vi "Rename Item Name.vi"(8 "error in (no error)":errorcluster, 9 "ForceRename?(F)":bool, 10 "New Name":string, 11 "Item Reference in":T1 format="%.0x") -> (0 "error out":errorcluster, 2 "Request invalid?":bool, 3 "Item Reference out":T1 format="%.0x")   [LabVIEW 2013, in "Hierarchy Framework.lvlib" / "Item.lvclass"]
doc: "Applies a <B>New Name</B> to the item specified by <B>Item Reference in</B>. If the <B>New Name</B> you specify already exists in the same section, this VI does nothing and the <B>Request invalid?</B> indicator returns TRUE."
uses:
  Item.lvclass
  Ctls/Item Reference.ctl
  Generic/Generic.lvclass
  Section/Section.lvclass
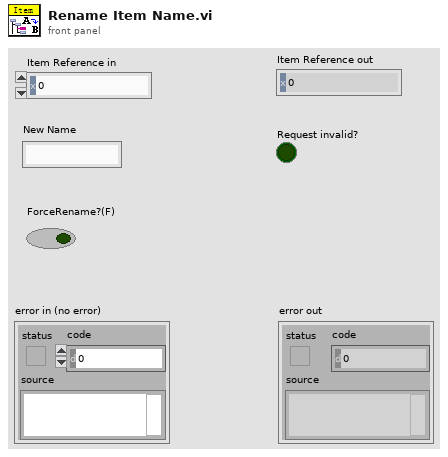
[diagram p1: front panel]
types:
  T1 = typedef "Hierarchy Framework.lvlib/Item.lvclass/Item Reference.ctl" = u64
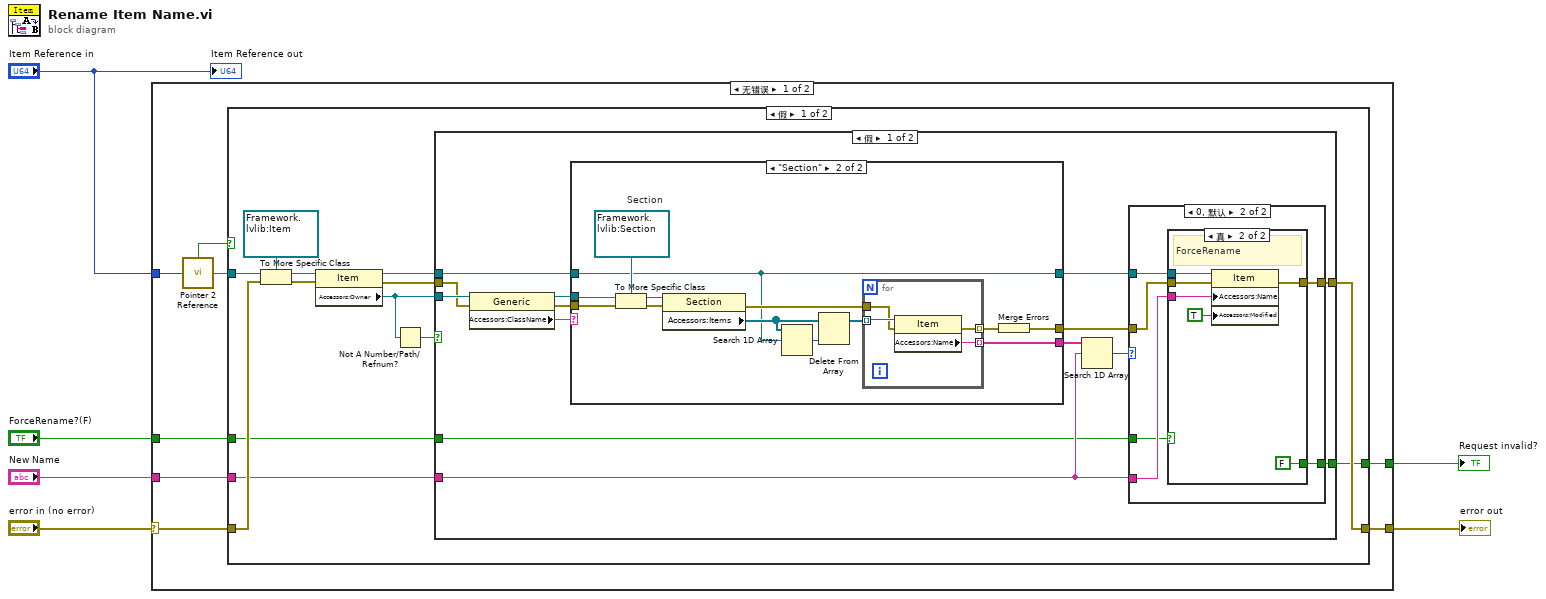
[diagram p0: block diagram]
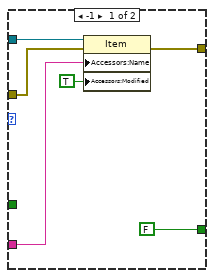
[diagram p2: hidden frame]
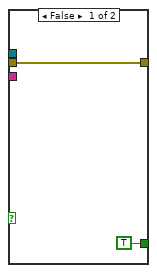
[diagram p3: hidden frame]
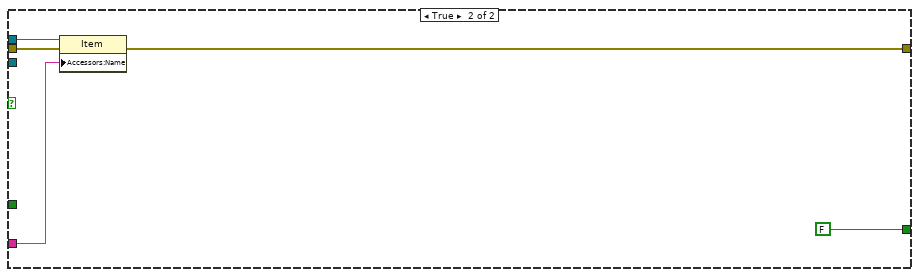
[diagram p5: hidden frame]
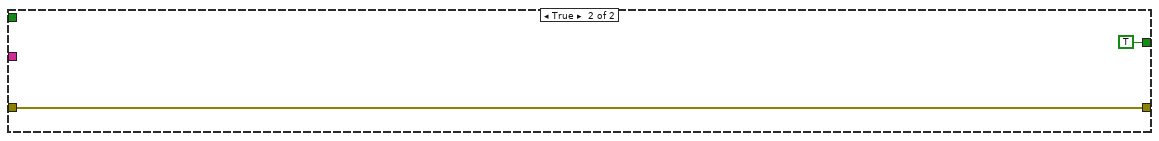
[diagram p6: hidden frame]
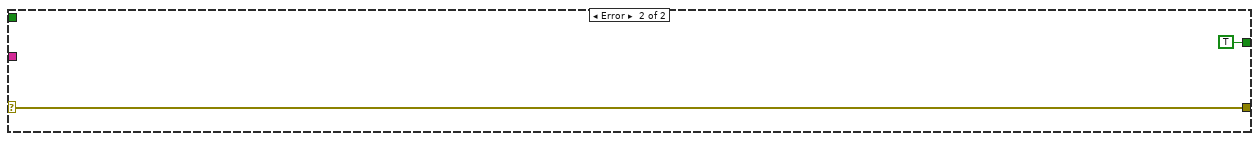
[diagram p7: hidden frame]
diagram:
  n1 = case shown="无错误" "error in (no error)" {
    selector: "error in (no error)" -> [w10 w89]
    tunnel: "Item Reference in" -> [w13 _]
    tunnel: "New Name" -> [w14 _]
    tunnel: [w9 w89] -> w4
    tunnel: [w8 TRUE] -> w2
    tunnel: "ForceRename?(F)" -> [w7 _]
    frame No Error {
      n2 = call "Pointer 2 Reference.vi"("Pointer"=w13) -> ("Not A Refnum?"=w12:bool, "Generic Reference"=w11:refnum<data-value>)
      n3 = case shown="假" w12 {
        tunnel: w11 -> [w27 _]
        tunnel: w14 -> [w18 _]
        tunnel: w10 -> [w25 w87]
        tunnel: [w17 w87] -> w9
        tunnel: [w16 TRUE] -> w8
        tunnel: w7 -> [w15 _]
        frame False {
          n4 = To More Specific Class(target class=refnum<data-value> refnum ("Item"), reference=w27, error in=w25) -> (specific class reference=w24:refnum<data-value>, error out=w23:errorcluster)
          n5 = property class="Item"(reference=w24, error in=w23) -> (reference out=w21:refnum<data-value>, error out=w20:errorcluster, "Accessors:Owner"=w19:refnum<data-value>)
          n6 = Not A Number/Path/Refnum?(number/path/refnum=w19) -> (NaN/Path/Refnum?=w22:bool)
          n7 = case shown="假" w22 {
            tunnel: w21 -> [w36 w85]
            tunnel: w20 -> [w40 w84]
            tunnel: w19 -> [w41 _]
            tunnel: w18 -> [w31 w83]
            tunnel: [w30 w82] -> w17
            tunnel: [w29 FALSE] -> w16
            tunnel: w15 -> [w28 _]
            frame False {
              n8 = property class="Generic"(reference=w41, error in=w40) -> (reference out=w38:refnum<data-value>, error out=w37:errorcluster, "Accessors:ClassName"=w39:string)
              n9 = case shown="\"Section\"" w39 {
                tunnel: w38 -> [_ w76]
                tunnel: w37 -> [w63 w75]
                tunnel: [_ w70] -> w35
                tunnel: [w63 w68] -> w32
                tunnel: w36 -> [w62 w64]
                tunnel: [w62 w64] -> w33
                frame "假", Default {
                }
                frame "Section" {
                  w74 = refnum<data-value> refnum  # Section
                  n10 = To More Specific Class(target class=w74, reference=w76, error in=w75) -> (specific class reference=w72:refnum<data-value>, error out=w73:errorcluster)
                  n11 = property class="Section"(reference=w72, error in=w73) -> (error out=w71:errorcluster, "Accessors:Items"=w67:refnum<data-value>[])  [unwired: 1 out]
                  n12 = Search 1D Array(1D array=w67, element=w64) -> (index of element=w65:i32)  [unwired: 1 in]
                  n13 = Delete From Array(array=w67, index=w65) -> (array with subset deleted=w66:refnum<data-value>[])  [unwired: 1 in, 1 out]
                  n14 = for {
                    tunnel: w66 -> [w80] mode=indexing
                    tunnel: w71 -> [w79]
                    tunnel: [w78] -> w69 mode=indexing
                    tunnel: [w77] -> w70 mode=indexing
                    n15 = property class="Item"(reference=w80, error in=w79) -> (error out=w78:errorcluster, "Accessors:Name"=w77:string)  [unwired: 1 out]
                  }
                  n16 = Merge Errors(w69) -> (w68:errorcluster)
                }
              }
              n17 = Search 1D Array(1D array=w35, element=w31) -> (index of element=w34:i32)  [unwired: 1 in]
              n18 = case shown="0, 默认" w34 {
                tunnel: w33 -> [w47 w53]
                tunnel: w32 -> [w46 w52]
                tunnel: w31 -> [w45 w51]
                tunnel: [w44 w50] -> w30
                tunnel: [FALSE w49] -> w29
                tunnel: w28 -> [_ w48]
                frame -1 {
                  n19 = property class="Item"(reference=w47, error in=w46, "Accessors:Name"=w45, "Accessors:Modified"=TRUE ("Modified")) -> (error out=w44:errorcluster)  [unwired: 1 out]
                }
                frame 0, Default {
                  n20 = case shown="真" w48 {
                    tunnel: w53 -> [_ w61]
                    tunnel: w52 -> [w55 w60]
                    tunnel: w51 -> [_ w59]
                    tunnel: [w55 w58] -> w50
                    tunnel: [TRUE FALSE] -> w49
                    frame False {
                    }
                    frame True {
                      # "ForceRename"
                      n21 = property class="Item"(reference=w61, error in=w60, "Accessors:Name"=w59, "Accessors:Modified"=TRUE ("Modified")) -> (error out=w58:errorcluster)  [unwired: 1 out]
                    }
                  }
                }
              }
            }
            frame True {
              n22 = property class="Item"(reference=w85, error in=w84, "Accessors:Name"=w83) -> (error out=w82:errorcluster)  [unwired: 1 out]
            }
          }
        }
        frame True {
        }
      }
    }
    frame Error {
    }
  }
  "Request invalid?" <- w2
  "error out" <- w4
  "Item Reference out" <- "Item Reference in"
